vi "Reference Rectangle.vi"(8 "error in (no error)":errorcluster, 10 "My VI":string, 11 "Ref VI in":refnum<class "Ref VI.lvclass">) -> (0 "error out":errorcluster, 2 "Rectangle":T1)   [LabVIEW 2020, in "Panel.lvlib" / "Ref VI.lvclass"]
doc: "Returns the center point to use as a reference when positioning the window.\n\n----\nPlease see the following web address for additional documentation and tutorial information:\nhttp://www.mooregoodideas.com/mgi-panel-manager/\n\nAuthor: Derek Trepanier\n\nCopyright (c) 2018, Moore Good Ideas, Inc.\n\nAll rights reserved.\n\nRedistribution and use in source and binary forms, with or without modification, are permitted provided that the following conditions are met:\n\n * Redistributions of source code must retain the above copyright notice, this list of conditions and the following disclaimer.\n * Redistributions in binary form must reproduce the above copyright notice, this list of conditions and the following disclaimer in the documentation and/or other materials provided with the distribution.\n * Neither the name of Moore Good Ideas, Inc. nor the names of its contributors may be used to endorse or promote products derived from this software without specific prior written permission.\n\nTHIS SOFTWARE IS PROVIDED BY THE COPYRIGHT HOLDERS AND CONTRIBUTORS \"AS IS\" AND ANY EXPRESS OR IMPLIED WARRANTIES, INCLUDING, BUT NOT LIMITED TO, THE IMPLIED WARRANTIES OF MERCHANTABILITY AND FITNESS FOR A PARTICULAR PURPOSE ARE DISCLAIMED. IN NO EVENT SHALL THE COPYRIGHT OWNER OR CONTRIBUTORS BE LIABLE FOR ANY DIRECT, INDIRECT, INCIDENTAL, SPECIAL, EXEMPLARY, OR CONSEQUENTIAL DAMAGES (INCLUDING, BUT NOT LIMITED TO, PROCUREMENT OF SUBSTITUTE GOODS OR SERVICES; LOSS OF USE, DATA, OR PROFITS; OR BUSINESS INTERRUPTION) HOWEVER CAUSED AND ON ANY THEORY OF LIABILITY, WHETHER IN CONTRACT, STRICT LIABILITY, OR TORT (INCLUDING NEGLIGENCE OR OTHERWISE) ARISING IN ANY WAY OUT OF THE USE OF THIS SOFTWARE, EVEN IF ADVISED OF THE POSSIBILITY OF SUCH DAMAGE."
uses:
  <vilib>/MGI/Panel Manager/Panel/Window Position/Reference Position/Ref VI/Ref VI.lvclass
  <vilib>/Utility/miscctls.llb/LVRectTypeDef.ctl
  <vilib>/MGI/Panel Manager/Panel/Window Position/Reference Position/Ref VI/Ref VI.lvclass/Ref VI.ctl
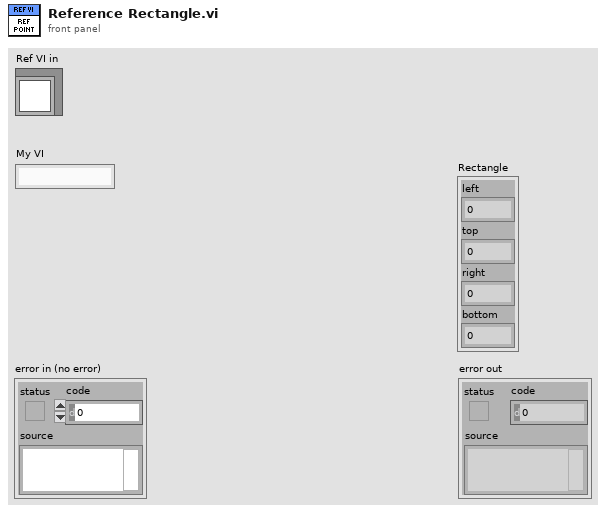
[diagram p1: front panel]
types:
  T1 = cluster{"left":i16, "top":i16, "right":i16, "bottom":i16}
  T2 = typedef "LVRectTypeDef.ctl" = cluster{"Left":i16, "Top":i16, "Right":i16, "Bottom":i16}
  T3 = enum32{"Invalid", "Standard", "Closed", "Hidden", "Minimized", "Maximized"}[]
  T4 = enum32{"Invalid", "Standard", "Closed", "Hidden", "Minimized", "Maximized"}
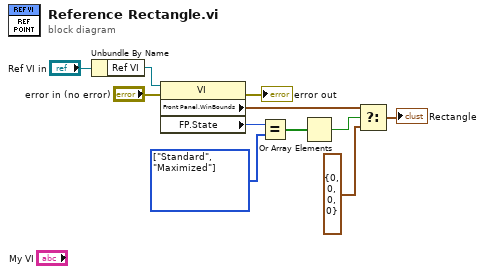
[diagram p0: block diagram]
diagram:
  w7 = T3 [enum."Standard", enum."Maximized"] items=["Invalid", "Standard", "Closed", "Hidden", "Minimized", "Maximized"]
  n1 = Unbundle By Name("Ref VI in") -> ("Ref VI"=w10:refnum<vi>)
  n2 = property class="VI"(reference=w10, error in="error in (no error)") -> (error out=→"error out":errorcluster, "Front Panel.WinBounds"=w3:T2, "FP.State"=w6:T4)  [unwired: 1 out]
  n3 = Equal?(x=w6, y=w7) -> (x = y?=w5:bool[])
  n4 = Or Array Elements(Boolean array=w5) -> (logical OR=w4:bool)
  n5 = Select(t=w3, s=w4, f=T2 {"Left"=0, "Top"=0, "Right"=0, "Bottom"=0}) -> (s? t:f=→"Rectangle":T2)
